vi "FGV_logger.vi"(8 "error in":errorcluster, 9 "?":T1={"Column"=-1, "Data"=""}, 11 "Command":enum16{"Update", "Log", "Init"}(ring)) -> (0 "error out":errorcluster)   [LabVIEW 2016]
uses:
  Typedef/LogInput.ctl
  <vilib>/Utility/file.llb/Write Delimited Spreadsheet (string).vi
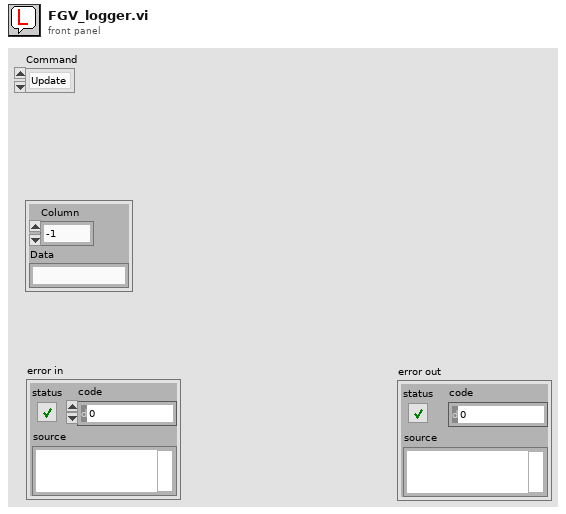
[diagram p1: front panel]
types:
  T1 = typedef "LogInput.ctl" = cluster{"Column":i32, "Data":string}
  T2 = enum16{"open", "replace", "create", "open or create", "replace or create", "replace or create with confirmation"}
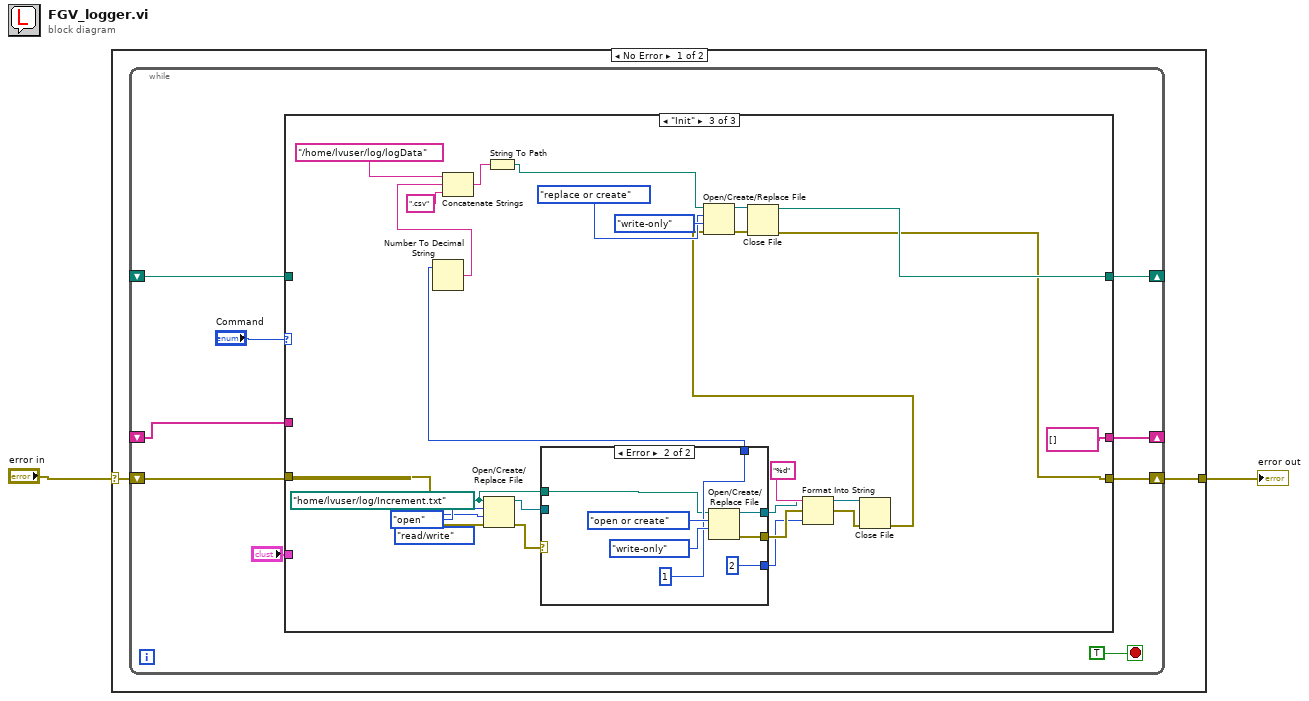
[diagram p0: block diagram]
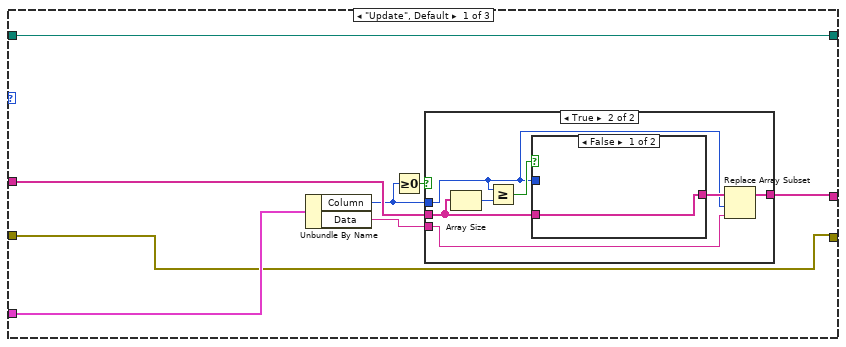
[diagram p2: hidden frame]
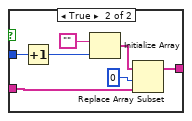
[diagram p4: hidden frame]
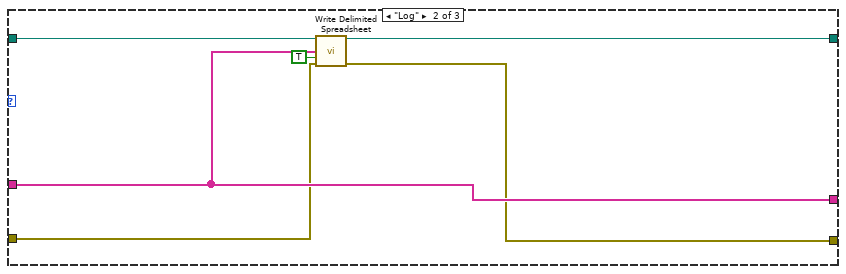
[diagram p5: hidden frame]
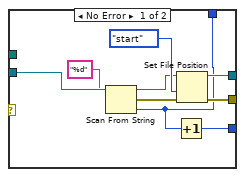
[diagram p6: hidden frame]
diagram:
  n1 = case shown="No Error" "error in" {
    selector: "error in" -> [w4 w86]
    tunnel: [w3 w86] -> w1
    frame No Error {
      n2 = while {
        shift-right: [w10] -> _
        shift-left: _ -> [w9]
        shift-right: [w7] -> w3
        shift-left: w4 -> [w8]
        shift-right: [w6] -> _
        shift-left: _ -> [w5]
        stop <- TRUE stop-if-true
        n3 = case shown="\"Init\"" "Command" {
          tunnel: "?" -> [w21 _ _]
          tunnel: [w18 w43 string[] []] -> w10
          tunnel: w9 -> [w20 w43 _]
          tunnel: w8 -> [w17 w39 w64]
          tunnel: [w17 w38 w48] -> w7
          tunnel: [w14 w42 w49] -> w6
          tunnel: w5 -> [w14 w41 _]
          frame "Update", Default {
            n4 = Unbundle By Name(w21) -> ("Column"=w15:i32, "Data"=w19:string)
            n5 = Greater Or Equal To 0?(x=w15) -> (x >= 0?=w16:bool)
            n6 = case shown="True" w16 {
              tunnel: w20 -> [w22 w27]
              tunnel: w19 -> [_ w25]
              tunnel: [w22 w24] -> w18
              tunnel: w15 -> [_ w23]
              frame False {
              }
              frame True {
                n7 = Array Size(array=w27) -> (size(s)=w29:i32)
                n8 = Greater Or Equal?(x=w23, y=w29) -> (x >= y?=w28:bool)
                n9 = case shown="False" w28 {
                  tunnel: w27 -> [w30 w32]
                  tunnel: [w30 w31] -> w26
                  tunnel: w23 -> [_ w36]
                  frame False {
                  }
                  frame True {
                    n10 = Increment(x=w36) -> (x+1=w35:i32)
                    n11 = Initialize Array("", w35) -> (w34:string[])
                    n12 = Replace Array Subset(array=w34, new element=w32, index=0) -> (w31:string[])
                  }
                }
                n13 = Replace Array Subset(array=w26, new element=w25, index=w23) -> (w24:string[])
              }
            }
          }
          frame "Log" {
            n14 = call-poly <vilib>:"Write Delimited Spreadsheet.vi"("file path (dialog if empty)"=w41, "1D data"=w43, "append to file? (new file:F)"=TRUE, "error in (no error)"=w39) -> ("new file path (Not A Path if cancelled)"=w42:path, "error out"=w38:errorcluster)  [unwired: 10 in]
          }
          frame "Init" {
            w44 = path "/home/lvuser/log/Increment.txt" ("file path (use dialog)")
            n15 = Open/Create/Replace File(file path (use dialog)=w44, error in=w64, operation (0:open)=T2."open", access (0:read/write)=enum16{"read/write", "read-only", "write-only"}."read/write") -> (refnum out=w63:refnum<file>, error out=w45:errorcluster)  [unwired: 2 in, 1 out]
            n16 = case shown="Error" w45 {
              tunnel: w63 -> [w78 _]
              tunnel: [w74 w80] -> w61
              tunnel: [w73 w81] -> w60
              tunnel: [w71 2] -> w59
              tunnel: [w70 1] -> w53
              tunnel: w44 -> [_ w79]
              frame No Error {
                n17 = Scan From String("%d" ("format string"), w78) -> (w75:refnum<file>, w72:errorcluster, output 1=w70:i32)  [unwired: 2 in]
                n18 = Increment(x=w70) -> (x+1=w71:i32)
                n19 = Set File Position(refnum=w75, from (0:start)=enum16{"start", "end", "current"}."start", error in=w72) -> (refnum out=w74:refnum<file>, error out=w73:errorcluster)  [unwired: 1 in]
              }
              frame Error {
                n20 = Open/Create/Replace File(file path (use dialog)=w79, operation (0:open)=T2."open or create", access (0:read/write)=enum16{"read/write", "read-only", "write-only"}."write-only") -> (refnum out=w80:refnum<file>, error out=w81:errorcluster)  [unwired: 3 in, 1 out]
              }
            }
            n21 = Number To Decimal String(number=w53) -> (decimal integer string=w52:string)  [unwired: 1 in]
            n22 = Concatenate Strings("/home/lvuser/log/logData" ("string"), w52, ".csv" ("string")) -> (w55:string)
            n23 = String To Path(string=w55) -> (path=w54:path)
            n24 = Format Into String(format string="%d", initial string=w61, error in=w60, w59) -> (resulting string=w58:refnum<file>, error out=w57:errorcluster)
            n25 = Close File(refnum=w58, error in=w57) -> (error out=w56:errorcluster)  [unwired: 1 out]
            n26 = Open/Create/Replace File(file path (use dialog)=w54, error in=w56, operation (0:open)=T2."replace or create", access (0:read/write)=enum16{"read/write", "read-only", "write-only"}."write-only") -> (refnum out=w50:refnum<file>, error out=w51:errorcluster)  [unwired: 2 in, 1 out]
            n27 = Close File(refnum=w50, error in=w51) -> (path=w49:path, error out=w48:errorcluster)
          }
        }
      }
    }
    frame Error {
    }
  }
  "error out" <- w1
